vi "start.vi"(8 "error in (no error)":errorcluster, 11 "K2602 in":refnum<class "K2602.lvclass">) -> (0 "error out":errorcluster, 3 "K2602 out":refnum<class "K2602.lvclass">)   [LabVIEW 2011, in "Hardware.lvlib" / "Channels.lvlib" / "K2602.lvclass"]
doc: "Abstract Method\n\nStarts/Arms the AnalogOutput task. Normally the AnalogOutput device is configured to wait for a trigger signal, therefore, in this case the method Arms the device ready for recieving its trigger upon which it will start outputing immediately its data."
uses:
  K2602.lvclass
  K2602.lvclass/K2602.ctl
  <instrlib>/Keithley 2600 Series/Keithley 2600 Series.lvlib
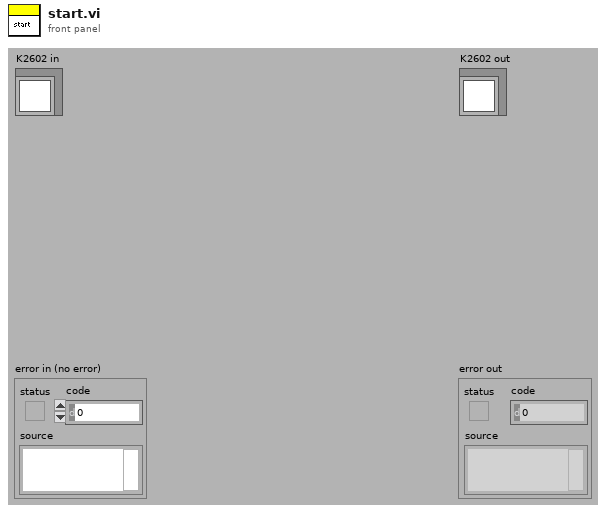
[diagram p1: front panel]
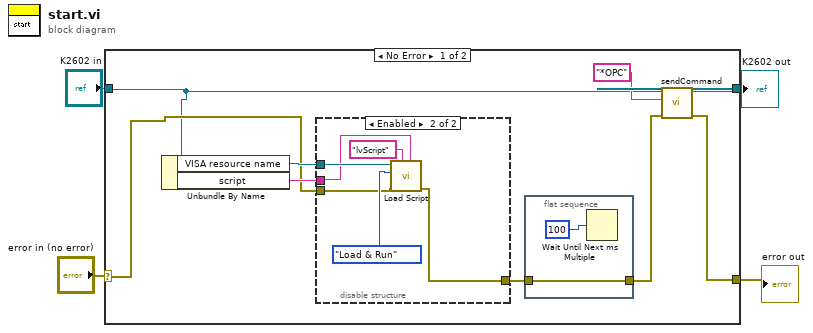
[diagram p0: block diagram]
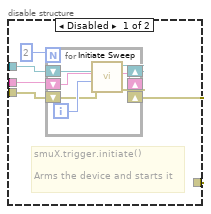
[diagram p2: hidden frame]
diagram:
  n1 = case shown="No Error" "error in (no error)" {
    selector: "error in (no error)" -> [w10 w34]
    tunnel: [w8 w35] -> w3
    tunnel: "K2602 in" -> [w9 w35]
    tunnel: [w7 w34] -> w1
    frame No Error {
      n2 = Unbundle By Name(w9) -> ("VISA resource name"=w12:refnum<visa-resource-name>, "script"=w13:string)
      n3 = disable-structure shown="Enabled" {
        disable-tunnel: w13 -> [w20 w30]
        disable-tunnel: w12 -> [w19 w33]
        disable-tunnel: w10 -> [w17 w31]
        disable-tunnel: [w16 w28] -> w5
        frame Disabled {
          # "smuX.trigger.initiate()\n\nArms the device and starts it"
          n4 = for {
            N: 2 -> [_]
            shift-right: [w22] -> _
            shift-left: w19 -> [w26]
            shift-right: [w21] -> _
            shift-left: w20 -> [w27]
            shift-right: [w23] -> w16
            shift-left: w17 -> [w24]
            i -> [w25]
            n5 = call <instrlib>:"Initiate Sweep.vi"("error in"=w24, "Channel (Channel A)"=w25, "Node In"=w27, "VISA resource name"=w26) -> ("error out"=w23:errorcluster, "Node Out"=w21:string, "VISA resource name out"=w22:refnum<visa-resource-name>)  [unwired: 4 in, 1 out]
          }
        }
        frame Enabled {
          n6 = call <instrlib>:"Load Script.vi"("Script"=w30, "Script Name"="lvScript", "error in"=w31, "Load Options (Load)"=enum16{"Load", "Load & Run"}."Load & Run", "VISA resource name"=w33) -> ("error out"=w28:errorcluster)  [unwired: 4 in, 2 out]
        }
      }
      n7 = flat-sequence {
        tunnel: [w14] -> w6
        tunnel: w5 -> [w14]
        frame #0 {
          n8 = Wait Until Next ms Multiple(millisecond multiple=100) -> ()  [unwired: 1 out]
        }
      }
      n9 = call "sendCommand.vi"("error in (no error)"=w6, "command"="*OPC", "K2602 in"=w9) -> ("error out"=w7:errorcluster, "K2602 out"=w8:refnum<class "K2602.lvclass">)  [unwired: 7 in]
    }
    frame Error {
    }
  }
  "error out" <- w1
  "K2602 out" <- w3
